vi "Add Points Double.vi"(7 "rebuild_threshold":sgl=1.0, 8 "error in (no error)":errorcluster, 10 "points":dbl[][](array[numeric]), 11 "KD Tree Double in":refnum<class "KD Tree Double.lvclass">) -> (0 "error out":errorcluster, 3 "KD Tree Double out":refnum<class "KD Tree Double.lvclass">)   [LabVIEW 2020, in "KD Tree.lvlib" / "KD Tree Double.lvclass"]
uses:
  KD Tree Double.lvclass
  KD Tree.lvlib
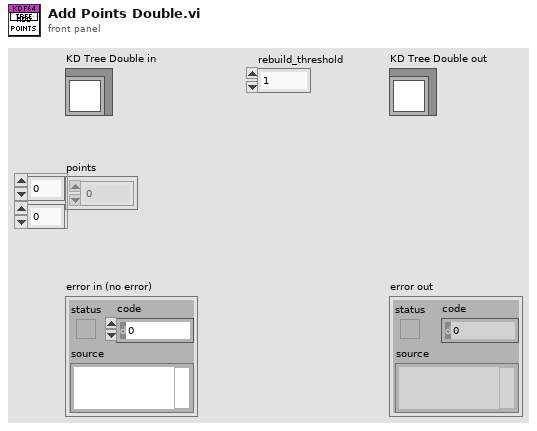
[diagram p1: front panel]
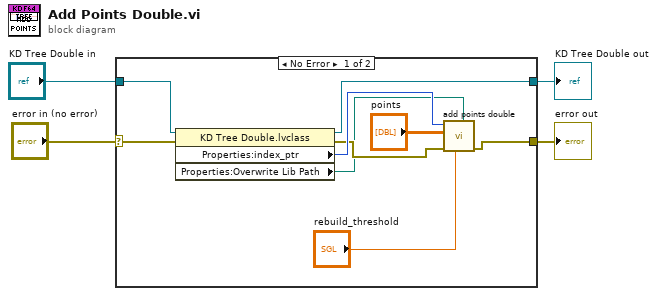
[diagram p0: block diagram]
diagram:
  n1 = case shown="No Error" "error in (no error)" {
    selector: "error in (no error)" -> [w13 w15]
    tunnel: [w5 w15] -> w3
    tunnel: [w11 w14] -> w1
    tunnel: "KD Tree Double in" -> [w12 w14]
    frame No Error {
      n2 = property class="KD Tree Double.lvclass"(reference=w12, error in=w13) -> (reference out=w11:refnum<class "KD Tree Double.lvclass">, error out=w8:errorcluster, "Properties:index_ptr"=w10:u64, "Properties:Overwrite Lib Path"=w6:path)
      n3 = call "add points double.vi"("Overwrite Lib Path"=w6, "rebuild_threshold"="rebuild_threshold", "error in (no error)"=w8, "points"="points", "index_ptr"=w10) -> ("error out"=w5:errorcluster)  [unwired: 5 in, 1 out]
    }
    frame Error {
    }
  }
  "error out" <- w3
  "KD Tree Double out" <- w1
